vi "Get All Exports.vi"(0 "Component in":refnum<class "Component.lvclass">) -> (4 "Component out":refnum<class "Component.lvclass">, 6 "Exports":refnum<class "Export.lvclass">[](array[class]))   [LabVIEW 2017, in "CL_G3_VIComponentBuilder.lvlib" / "Component.lvclass"]
doc: "Get's all of the exports defined by the component."
uses:
  Component.lvclass
  Exports/Exports/Export.lvclass
  Component.lvclass/Component.ctl
  Accessors/Write Component Operations Errors.vi
  Accessors/Read Component Operations Errors.vi
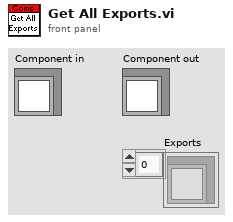
[diagram p1: front panel]
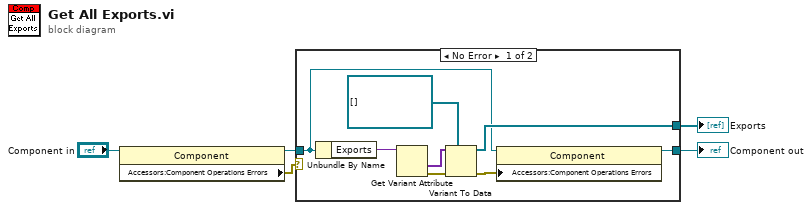
[diagram p0: block diagram]
diagram:
  n1 = property class="Component"(reference="Component in") -> (reference out=w2:refnum<class "Component.lvclass">, "Accessors:Component Operations Errors"=w1:errorcluster)  [unwired: 1 in, 1 out]
  n2 = case shown="No Error" w1 {
    tunnel: [w7 w14] -> w4
    tunnel: [w12 _] -> w5
    tunnel: w2 -> [w8 w14]
    frame No Error {
      n3 = Unbundle By Name(w8) -> ("Exports"=w11:variant)
      n4 = Get Variant Attribute(Variant=w11) -> (values=w10:variant[], error out=w9:errorcluster)  [unwired: 3 in, 2 out]
      n5 = Variant To Data(error in=w9, type=refnum<class "Export.lvclass">[] [], Variant=w10) -> (data=w12:refnum<class "Export.lvclass">[], error out=w6:errorcluster)
      n6 = property class="Component"(reference=w8, "Accessors:Component Operations Errors"=w6) -> (reference out=w7:refnum<class "Component.lvclass">)  [unwired: 1 in, 1 out]
    }
    frame Error {
    }
  }
  "Component out" <- w4
  "Exports" <- w5
